vi "signal_mapping_PMT-measurement_7_9.vi"() -> ()   [LabVIEW 2022 SP3]
uses:
  <vilib>/Analysis/1siggen.llb/Ramp Pattern by Samples.vi
  <vilib>/Utility/file.llb/Write Delimited Spreadsheet (string).vi
  <vilib>/Utility/file.llb/Write Delimited Spreadsheet (DBL).vi
  <vilib>/Analysis/NI_AALBase.lvlib
panel:
  out "y voltage":dbl=3.1578947368421053
  out "X voltage":dbl=6.947368421052631
  in  "IT":i32=200 caption="Set Gate Time (ms)"
  in  "RN":i32=2 caption="Set Gate Number"
  out "OVL":bool caption="LED ON : Over Rang Data"
  out "OLD":i32
  out "GN":i32=1 caption="Gate Number"
  out "DB":u32[](array[numeric])=[7, 0, 0, 0, 0, 0, 0, 0, 0, 0, 0, 0, 0, 0, 0, 0]
  out "Counts":i32[](array[numeric])=[4, 7]
  out "Handle Number":i32
  in  "Correction":bool=TRUE
  in  "max_step (V)":dbl=1.0 format="%#_13g"
  in  "ms to wait after move":u32=100
  in  "ANC300 address":refnum<visa-resource-name>="COM8"
  in  "Snake":bool
  in  "File to save to":path=path "D:/LabData/XiaoWang_Group_data_2024on/StackingTransitions/NbOI2/Lvgroup/samples/22p5deg/SHG/mapping_positions/mapping8_wp0.txt"
  in  "Select Scan Type":u16(ring)=1 items=["line scan", "rectangular scan"]
  in  "scan points":i32
  in  "y end":i32
  in  "x end":i32
  in  "y start":i32
  in  "x start":i32
  in  "y scan points":i32=20
  in  "x scan points":i32=20
  in  "y scan size":i32=12
  in  "x scan size":i32=12
  in  "y center":i32=6
  in  "x center":i32=6
  # "Scaning Setup"
  # "Rectangular Scan Parameters"
  # "Line Scan Parameters"
  # "Measurement Setup"
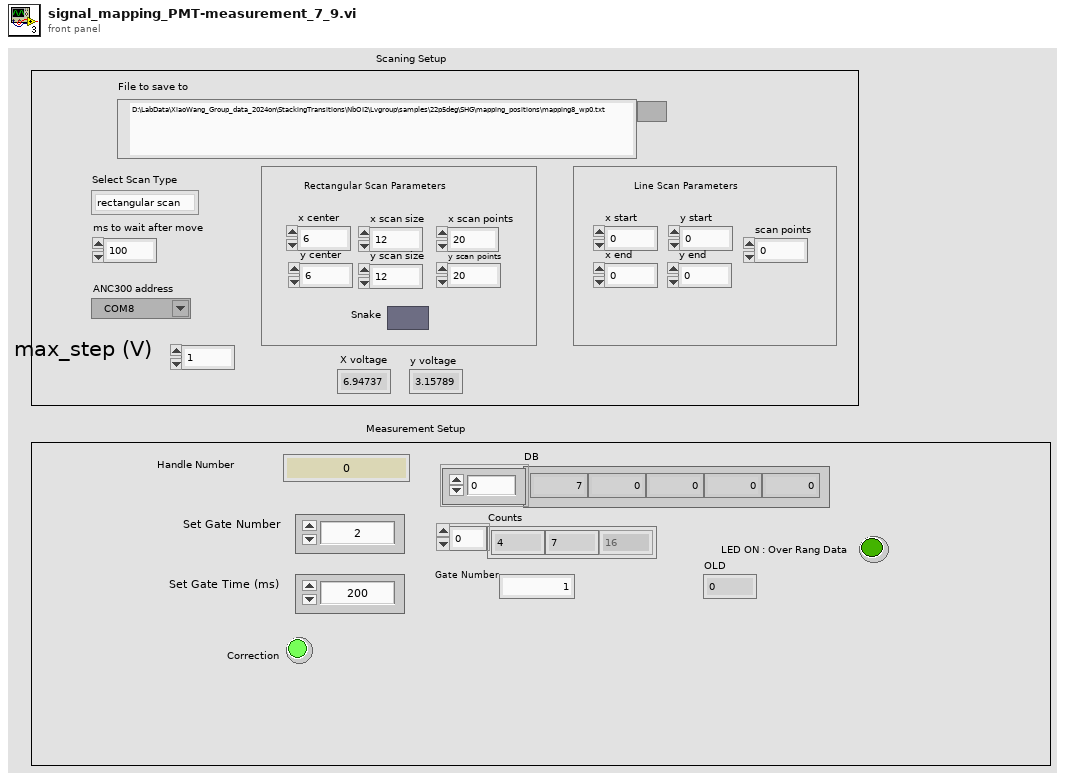
[diagram p1: front panel]
types:
  T1 = cluster{"error ":bool, "error number":i32, "error code":string}
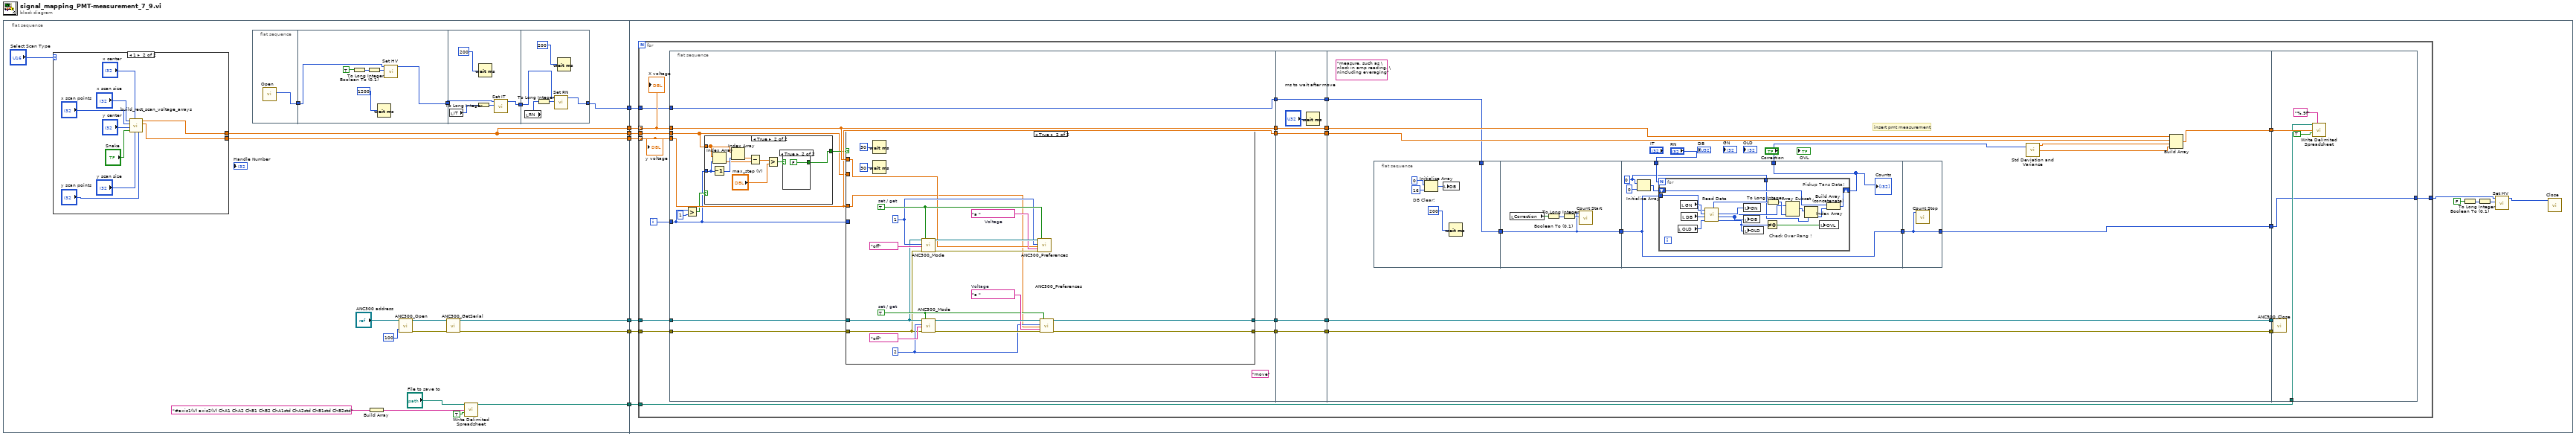
[diagram p0: block diagram]
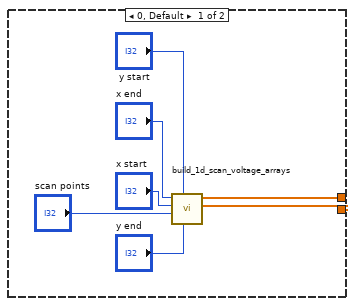
[diagram p2: hidden frame]
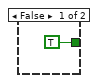
[diagram p3: hidden frame]
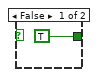
[diagram p4: hidden frame]
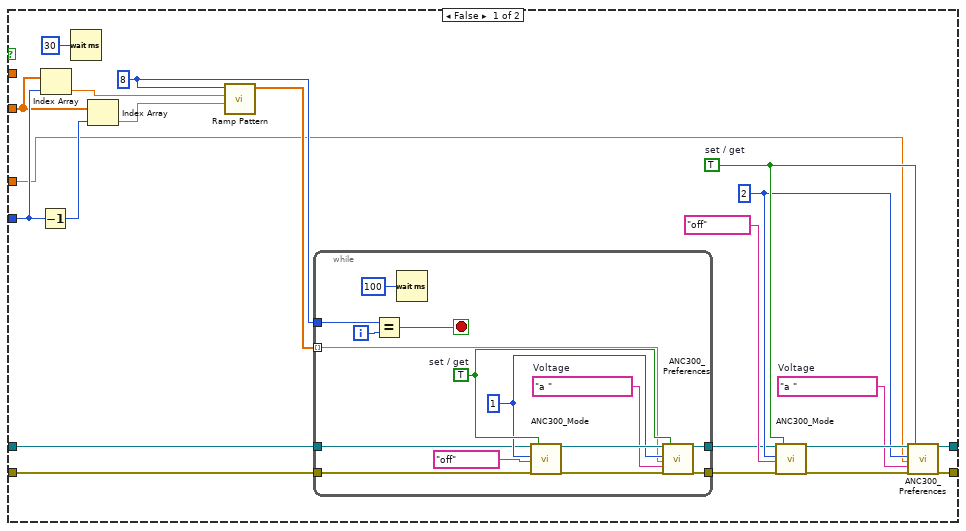
[diagram p5: hidden frame]
diagram:
  n1 = flat-sequence {
    tunnel: [w13] -> w7
    tunnel: [w25] -> w6
    tunnel: [w20] -> w5
    tunnel: [w19] -> w4
    tunnel: [w12] -> w3
    tunnel: [w13] -> w2
    tunnel: [w11] -> w1
    tunnel: w7 -> [w70]
    tunnel: w6 -> [w69]
    tunnel: w5 -> [w68]
    tunnel: w4 -> [w67]
    tunnel: w3 -> [w66]
    tunnel: w2 -> [w65]
    tunnel: w1 -> [w64]
    frame #0 {
      n2 = case shown="1" "Select Scan Type" {
        tunnel: [w43 w58] -> w25
        tunnel: [w44 w57] -> w13
        frame 0, Default {
          n3 = call "build_1d_scan_voltage_arrays.vi"("y end"="y end", "y start"="y start", "scan points"="scan points", "x start"="x start", "x end"="x end") -> ("y voltage array"=w43:dbl[], "x voltage array"=w44:dbl[])  [unwired: 5 in]
        }
        frame 1 {
          n4 = call "build_rect_scan_voltage_arrays.vi"("y scan points"="y scan points", "y scan size"="y scan size", "x center"="x center", "Snake"="Snake", "y center"="y center", "x scan points"="x scan points", "x scan size"="x scan size") -> ("y voltage array"=w58:dbl[], "x voltage array"=w57:dbl[])  [unwired: 3 in]
        }
      }
      n5 = flat-sequence {
        tunnel: [w26] -> w9
        tunnel: w9 -> [w27]
        tunnel: [w28] -> w8
        tunnel: w8 -> [w34]
        tunnel: [w35] -> w10
        tunnel: [w41] -> w11
        tunnel: w10 -> [w40]
        frame #0 {
          n6 = call "Open.vi"() -> ("Handle Number"=w26:i32)  [unwired: 10 in, 1 out]
        }
        frame #1 {
          n7 = Boolean To (0,1)(Boolean=TRUE) -> (0, 1=w31:i16)
          n8 = To Long Integer(number=w31) -> (32bit integer=w32:i32)
          n9 = Wait (ms)(milliseconds to wait=u32 1200) -> ()  [unwired: 1 out]
          n10 = call "Set HV.vi"("HV"=w32, "handle"=w27) -> ("handle out"=w28:i32)  [unwired: 8 in, 1 out]
        }
        frame #2 {
          n11 = local read "IT"() -> (w33:i32)
          n12 = To Long Integer(number=w33) -> (32bit integer=w37:i32)
          n13 = Wait (ms)(milliseconds to wait=u32 200) -> ()  [unwired: 1 out]
          n14 = call "Set IT.vi"("IT"=w37, "handle"=w34) -> ("handle out"=w35:i32)  [unwired: 8 in, 1 out]
        }
        frame #3 {
          n15 = local read "RN"() -> (w39:i32)
          n16 = To Long Integer(number=w39) -> (32bit integer=w42:i32)
          n17 = call "Set RN.vi"("RN"=w42, "handle"=w40) -> ("handle out"=w41:i32)  [unwired: 8 in, 1 out]
          n18 = Wait (ms)(milliseconds to wait=u32 200) -> ()  [unwired: 1 out]
        }
      }
      n19 = Build Array("#axis1(V) axis2(V) ChA1 ChA2 ChB1 ChB2 ChA1std ChA2std ChB1std ChB2std") -> (w15:string[])
      n20 = call "ANC300_Open.vi"("ANC300 Communication Port In"="ANC300 address", "milliseconds to wait"=u32 100 ("millisecond timer value")) -> ("ANC300 Communication Port Out"=w21:refnum<visa-resource-name>, "error out"=w18:T1)  [unwired: 13 in, 3 out]
      n21 = call "ANC300_GetSerial.vi"("ANC300 Communication Port In"=w21, "error in"=w18) -> ("ANC300 Communication Port Out"=w20:refnum<visa-resource-name>, "error out"=w19:T1)  [unwired: 10 in, 6 out]
      n22 = call-poly <vilib>:"Write Delimited Spreadsheet.vi"("file path (dialog if empty)"="File to save to", "1D data"=w15, "append to file? (new file:F)"=TRUE) -> ("new file path (Not A Path if cancelled)"=w12:path)  [unwired: 11 in, 1 out]
    }
    frame #1 {
      n23 = for {
        tunnel: w70 -> [w93] mode=indexing
        tunnel: w69 -> [w92] mode=indexing
        tunnel: w68 -> [w91]
        tunnel: w67 -> [w90]
        tunnel: w66 -> [w84]
        tunnel: w65 -> [w77]
        tunnel: w64 -> [w72]
        tunnel: [w71] -> w60
        i -> [w76]
        n24 = flat-sequence {
          tunnel: w93 -> [w103]
          tunnel: w92 -> [w102]
          tunnel: w91 -> [w105]
          tunnel: w90 -> [w104]
          tunnel: [w103] -> w87
          tunnel: [w102] -> w86
          tunnel: [w95] -> w83
          tunnel: [w96] -> w80
          tunnel: w77 -> [w98]
          tunnel: w76 -> [w97]
          tunnel: [w94] -> w73
          tunnel: w72 -> [w94]
          tunnel: [w178] -> w88
          tunnel: w87 -> [w178]
          tunnel: w86 -> [w177]
          tunnel: [w177] -> w85
          tunnel: w83 -> [w176]
          tunnel: [w176] -> w82
          tunnel: [w175] -> w81
          tunnel: w80 -> [w175]
          tunnel: [w174] -> w74
          tunnel: w73 -> [w174]
          tunnel: [w193] -> w89
          tunnel: w88 -> [w192]
          tunnel: w85 -> [w191]
          tunnel: w82 -> [w190]
          tunnel: w81 -> [w189]
          tunnel: [w190] -> w79
          tunnel: [w189] -> w78
          tunnel: [w187] -> w75
          tunnel: w74 -> [w186]
          tunnel: w89 -> [w230]
          tunnel: w84 -> [w228]
          tunnel: w79 -> [w227]
          tunnel: w78 -> [w226]
          tunnel: w75 -> [w225]
          tunnel: [w225] -> w71
          frame #0 {
            (unwired) "move"
            n25 = Greater?(x=w97, y=1) -> (0:w101:bool)
            n26 = case shown="True" w101 {
              tunnel: w98 -> [_ w115]
              tunnel: w97 -> [_ w114]
              tunnel: [TRUE w107] -> w99
              frame False {
              }
              frame True {
                n27 = Decrement(x=w114) -> (x-1=w113:i32)
                n28 = Index Array(array=w115, index=w114) -> (element=w112:dbl)
                n29 = Index Array(array=w115, index=w113) -> (element=w111:dbl)
                n30 = Subtract(x=w111, y=w112) -> (x-y=w110:dbl)
                n31 = Greater?(x=w110, y="max_step (V)") -> (0:w108:bool)
                n32 = case shown="True" w108 {
                  tunnel: [TRUE FALSE] -> w107
                  frame False {
                  }
                  frame True {
                  }
                }
              }
            }
            n33 = case shown="True" w99 {
              tunnel: w105 -> [w132 w160]
              tunnel: w104 -> [w131 w159]
              tunnel: w103 -> [_ w157]
              tunnel: w102 -> [w118 w156]
              tunnel: w98 -> [w136 _]
              tunnel: w97 -> [w138 _]
              tunnel: [w120 w154] -> w96
              tunnel: [w119 w155] -> w95
              frame False {
                w124 = 2
                w125 = TRUE  # set / get
                w127 = "a "  # Voltage
                w130 = 8
                n34 = Decrement(x=w138) -> (x-1=w137:i32)
                n35 = Index Array(array=w136, index=w138) -> (element=w135:dbl)
                n36 = Wait (ms)(milliseconds to wait=u32 30 ("2: ms to wait")) -> ()  [unwired: 1 out]
                n37 = Index Array(array=w136, index=w137) -> (element=w134:dbl)
                n38 = call-poly <vilib>:"Ramp Pattern.vi"("start"=w134, "end"=w135, "samples"=w130) -> ("Ramp Pattern"=w133:dbl[])  [unwired: 7 in, 1 out]
                n39 = while {
                  tunnel: w133 -> [w144] mode=indexing
                  tunnel: w132 -> [w146]
                  tunnel: w131 -> [w145]
                  tunnel: w130 -> [w142]
                  tunnel: [w140] -> w122
                  tunnel: [w139] -> w121
                  i -> [w143]
                  stop <- w141 stop-if-true
                  w147 = 1
                  w148 = TRUE  # set / get
                  w151 = "a "  # Voltage
                  n40 = Equal?(x=w142, y=w143) -> (x = y?=w141:bool)
                  n41 = Wait (ms)(milliseconds to wait=u32 100 ("1: ms to wait")) -> ()  [unwired: 1 out]
                  n42 = call "ANC300_Mode.vi"("ANC300 Communication Port In"=w146, "Axis"=w147, "axis mode in"="off", "error in"=w145, "set / get"=w148) -> ("ANC300 Communication Port Out"=w153:refnum<visa-resource-name>, "error out"=w152:T1)  [unwired: 8 in, 5 out]
                  n43 = call "ANC300_Preferences.vi"("ANC300 Communication Port In"=w153, "Axis"=w147, "value in"=w144, "parameter"=w151, "error in"=w152, "set / get"=w148) -> ("ANC300 Communication Port Out"=w140:refnum<visa-resource-name>, "error out"=w139:T1)  [unwired: 6 in, 6 out]
                }
                n44 = call "ANC300_Mode.vi"("ANC300 Communication Port In"=w122, "Axis"=w124, "axis mode in"="off", "error in"=w121, "set / get"=w125) -> ("ANC300 Communication Port Out"=w129:refnum<visa-resource-name>, "error out"=w128:T1)  [unwired: 8 in, 5 out]
                n45 = call "ANC300_Preferences.vi"("ANC300 Communication Port In"=w129, "Axis"=w124, "value in"=w118, "parameter"=w127, "error in"=w128, "set / get"=w125) -> ("ANC300 Communication Port Out"=w119:refnum<visa-resource-name>, "error out"=w120:T1)  [unwired: 6 in, 6 out]
              }
              frame True {
                w161 = 2
                w162 = 1
                w163 = TRUE  # set / get
                w165 = "a "  # Voltage
                w168 = TRUE  # set / get
                w171 = "a "  # Voltage
                n46 = Wait (ms)(milliseconds to wait=u32 30 ("2: ms to wait")) -> ()  [unwired: 1 out]
                n47 = Wait (ms)(milliseconds to wait=u32 30 ("1: ms to wait")) -> ()  [unwired: 1 out]
                n48 = call "ANC300_Mode.vi"("ANC300 Communication Port In"=w160, "Axis"=w162, "axis mode in"="off", "error in"=w159, "set / get"=w168) -> ("ANC300 Communication Port Out"=w173:refnum<visa-resource-name>, "error out"=w172:T1)  [unwired: 8 in, 5 out]
                n49 = call "ANC300_Mode.vi"("ANC300 Communication Port In"=w160, "Axis"=w161, "axis mode in"="off", "error in"=w159, "set / get"=w163) -> ("ANC300 Communication Port Out"=w167:refnum<visa-resource-name>, "error out"=w166:T1)  [unwired: 8 in, 5 out]
                n50 = call "ANC300_Preferences.vi"("ANC300 Communication Port In"=w173, "Axis"=w162, "value in"=w157, "parameter"=w171, "error in"=w172, "set / get"=w168) -> ()  [unwired: 6 in, 8 out]
                n51 = call "ANC300_Preferences.vi"("ANC300 Communication Port In"=w167, "Axis"=w161, "value in"=w156, "parameter"=w165, "error in"=w166, "set / get"=w163) -> ("ANC300 Communication Port Out"=w155:refnum<visa-resource-name>, "error out"=w154:T1)  [unwired: 6 in, 6 out]
              }
            }
          }
          frame #1 {
            n52 = Wait (ms)(milliseconds to wait="ms to wait after move") -> ()  [unwired: 1 out]
          }
          frame #2 {
            (unwired) "measure, such as \nlock in amp reading, \nincluding everaging"
            # "insert pmt measurement"
            n53 = flat-sequence {
              tunnel: [w194] -> w180
              tunnel: w186 -> [w194]
              tunnel: [w199] -> w188
              tunnel: w180 -> [w199]
              tunnel: [w208] -> w185
              tunnel: w188 -> [w208]
              tunnel: [w207] -> w183
              tunnel: "RN" -> [w206]
              tunnel: w185 -> [w224]
              tunnel: [w224] -> w187
              frame #0 {
                # "DB Clear!"
                n54 = Initialize Array(u32 0, 16 ("次元サイズ")) -> (w198:u32[])
                n55 = local write "DB"(w198) -> ()
                n56 = Wait (ms)(milliseconds to wait=u32 200) -> ()  [unwired: 1 out]
              }
              frame #1 {
                n57 = local read "Correction"() -> (w202:bool)
                n58 = Boolean To (0,1)(Boolean=w202) -> (0, 1=w200:i16)
                n59 = To Long Integer(number=w200) -> (32bit integer=w201:i32)
                n60 = call "Count Start.vi"("Correction"=w201, "handle"=w199) -> ()  [unwired: 8 in, 2 out]
              }
              frame #2 {
                w203 = u32 0
                n61 = Initialize Array(w203, 0 ("次元サイズ")) -> (w204:u32[])
                n62 = for {
                  N: w206 -> [_]
                  tunnel: w208 -> [w214]
                  shift-right: [w212] -> w207
                  shift-left: w204 -> [w213]
                  tunnel: w203 -> [w210]
                  # "Check Over Rang !"
                  # "Pickup Tans Data!"
                  n63 = local read "OLD"() -> (w223:i32)
                  n64 = local read "GN"() -> (w221:i32)
                  n65 = local read "DB"() -> (w222:u32[])
                  n66 = call "Read Data.vi"("OLD"=w223, "DataBuf"=w222, "GateNum"=w221, "handle"=w214) -> ("OLD out"=w216:i32, "DataBuf out"=w215:u32[], "GateNum out"=w217:i32, "function return"=w218:u32)  [unwired: 3 in, 1 out]
                  n67 = local write "GN"(w217) -> ()
                  n68 = local write "DB"(w215) -> ()
                  n69 = local write "OLD"(w216) -> ()
                  n70 = Not Equal To 0?(x=w216) -> (x != 0?=w220:bool)
                  n71 = To Long Integer(number=w218) -> (32bit integer=w219:i32)
                  n72 = Array Subset(array=w215, length=w219) -> (w211:u32[])  [unwired: 1 in]
                  n73 = Index Array(array=w211, index=w210) -> (element=w209:u32)
                  n74 = local write "OVL"(w220) -> ()
                  n75 = Build Array (concatenate)(w213, w209) -> (w212:u32[])
                }
                "Counts" <- w207
              }
              frame #3 {
                n76 = call "Count Stop.vi"("handle"=w224) -> ()  [unwired: 9 in, 2 out]
              }
            }
            n77 = call <vilib>:"Std Deviation and Variance.vi"("X"=w183) -> ("mean"=w182:dbl, "standard deviation"=w181:dbl)  [unwired: 1 in, 1 out]
            n78 = Build Array(w192, w191, w182, w181) -> (w193:dbl[])
          }
          frame #3 {
            n79 = call "ANC300_Close.vi"("ANC300 Communication Port In"=w227, "error in"=w226) -> ()  [unwired: 17 in, 1 out]
            n80 = call-poly <vilib>:"Write Delimited Spreadsheet.vi"("file path (dialog if empty)"=w228, "format (%.3f)"="%.9f", "1D data"=w230, "append to file? (new file:F)"=TRUE) -> ()  [unwired: 10 in, 2 out]
          }
        }
        "X voltage" <- w93
        "y voltage" <- w92
      }
      n81 = Boolean To (0,1)(Boolean=FALSE) -> (0, 1=w62:i16)
      n82 = To Long Integer(number=w62) -> (32bit integer=w63:i32)
      n83 = call "Set HV.vi"("HV"=w63, "handle"=w60) -> ("handle out"=w59:i32)  [unwired: 8 in, 1 out]
      n84 = call "Close.vi"("Handle"=w59) -> ()  [unwired: 9 in, 2 out]
    }
  }
